vi "FG_NamedQueues.vi"(7 "action":T1, 8 "error in":errorcluster, 10 "queues in":refnum<class "CLM_PriorityLocalMessage.lvclass">, 11 "name":string) -> (0 "error out":errorcluster, 1 "failed?":bool, 2 "queues out":refnum<class "CLM_PriorityLocalMessage.lvclass">)   [LabVIEW 2013, in "CLM_PriorityLocalMessage.lvclass"]
uses:
  CLM_PriorityLocalMessage.lvclass
  FG_NamedQueuesAction.ctl
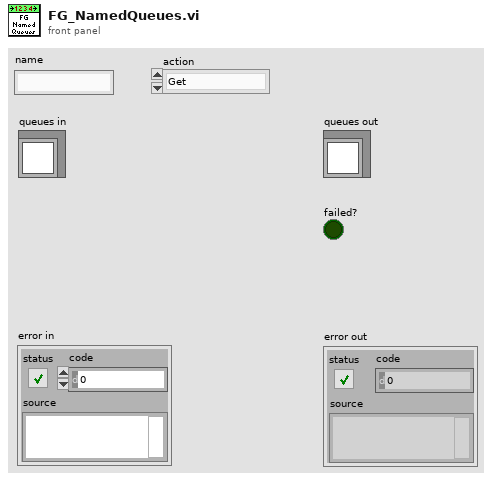
[diagram p1: front panel]
types:
  T1 = typedef "CLM_PriorityLocalMessage.lvclass/FG_NamedQueuesAction.ctl" = enum16{"Get", "Add", "Remove", "RemoveAll"}
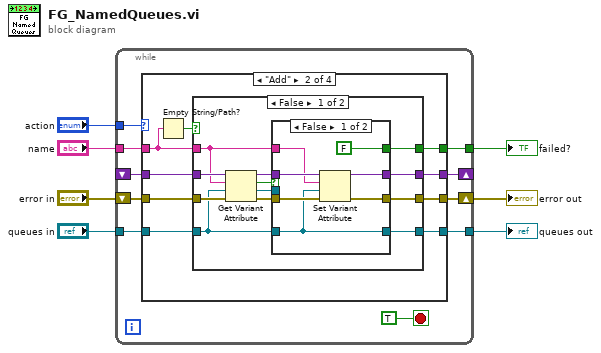
[diagram p0: block diagram]
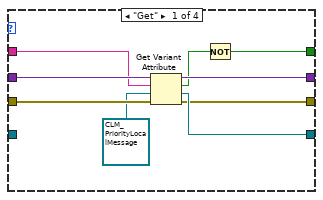
[diagram p2: hidden frame]
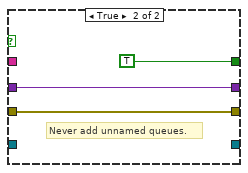
[diagram p4: hidden frame]
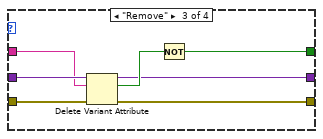
[diagram p5: hidden frame]
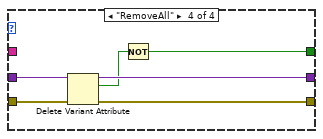
[diagram p6: hidden frame]
diagram:
  n1 = while {
    tunnel: "action" -> [w17]
    tunnel: "name" -> [w16]
    shift-right: [w15] -> _
    shift-left: _ -> [w14]
    tunnel: [w13] -> w5
    tunnel: [w12] -> w4
    shift-right: [w11] -> w3
    shift-left: "error in" -> [w10]
    tunnel: "queues in" -> [w8]
    stop <- TRUE stop-if-true
    n2 = case shown="\"Add\"" w17 {
      tunnel: w16 -> [w20 w28 w66 _]
      tunnel: [w26 w32 w64 w71] -> w15
      tunnel: w14 -> [w25 w35 w68 w74]
      tunnel: [w21 w33 w62 w69] -> w13
      tunnel: [w24 w30 _ _] -> w12
      tunnel: [w23 w31 w63 w72] -> w11
      tunnel: w10 -> [w22 w34 w67 w73]
      tunnel: w8 -> [_ w29 _ _]
      frame "Get" {
        n3 = Get Variant Attribute(Variant=w25, name=w20, default value (empty Variant)=refnum<class "CLM_PriorityLocalMessage.lvclass"> refnum ("NISE_PriorityLocalMessage.lvclass"), error in=w22) -> (duplicate Variant=w26:variant, found=w18:bool, value=w24:refnum<class "CLM_PriorityLocalMessage.lvclass">, error out=w23:errorcluster)
        n4 = Not(x=w18) -> (.not. x?=w21:bool)
      }
      frame "Add" {
        n5 = Empty String/Path?(string/path=w28) -> (empty?=w27:bool)
        n6 = case shown="False" w27 {
          tunnel: w35 -> [w47 w60]
          tunnel: w34 -> [w46 w59]
          tunnel: [w44 TRUE] -> w33
          tunnel: [w42 w60] -> w32
          tunnel: [w40 w59] -> w31
          tunnel: [w38 _] -> w30
          tunnel: w29 -> [w37 _]
          tunnel: w28 -> [w36 _]
          frame False {
            n7 = Get Variant Attribute(Variant=w47, name=w36, default value (empty Variant)=w37, error in=w46) -> (duplicate Variant=w43:variant, found=w45:bool, value=w39:refnum<class "CLM_PriorityLocalMessage.lvclass">, error out=w41:errorcluster)
            n8 = case shown="False" w45 {
              selector: w45 -> [_ w58]
              tunnel: [FALSE w58] -> w44
              tunnel: w43 -> [w54 w57]
              tunnel: [w50 w57] -> w42
              tunnel: w41 -> [w53 w56]
              tunnel: [w51 w56] -> w40
              tunnel: w39 -> [_ w55]
              tunnel: [w49 w55] -> w38
              tunnel: w36 -> [w52 _]
              tunnel: w37 -> [w49 _]
              frame False {
                n9 = Set Variant Attribute(Variant=w54, name=w52, value=w49, error in=w53) -> (Variant out=w50:variant, error out=w51:errorcluster)  [unwired: 1 out]
              }
              frame True {
              }
            }
          }
          frame True {
            # "Never add unnamed queues."
          }
        }
      }
      frame "Remove" {
        n10 = Delete Variant Attribute(4:w67, 6:w66, 7:w68) -> (0:w63:errorcluster, 2:w65:bool, 3:w64:variant)
        n11 = Not(x=w65) -> (.not. x?=w62:bool)
      }
      frame "RemoveAll" {
        n12 = Delete Variant Attribute(4:w73, 7:w74) -> (0:w72:errorcluster, 2:w70:bool, 3:w71:variant)  [unwired: 1 in]
        n13 = Not(x=w70) -> (.not. x?=w69:bool)
      }
    }
  }
  "error out" <- w3
  "failed?" <- w5
  "queues out" <- w4
